vi "parseRangeMode.vi"(8 "error in (no error)":errorcluster, 11 "String":string) -> (0 "error out":errorcluster, 3 "Data":dbl[](array[numeric]))   [LabVIEW 2023, in "CCD.lvclass"]
uses:
  CCD.lvclass
  8fe7bb78-7376-43c1-906c-2fa6ce8d17f9.vi
  <vilib>/JDP Science/JSONtext/Find Item.vi
  <vilib>/JDP Science/JSONtext/Next JSON Value.vi
  <vilib>/JDP Science/JSONtext/String Subset.vi
  <vilib>/JDP Science/JSONtext/Parsing/Advance past next JSON Value (inlined COPY).vi
  <vilib>/JDP Science/JSONtext/Parsing/Advance past whitespace.vi
  <vilib>/JDP Science/JSONtext/Parsing/Advance past String.vi
  <vilib>/JDP Science/JSONtext/Parsing/Advance past Number.vi
  <vilib>/JDP Science/JSONtext/Parsing/Advance past Line Ending.vi
  <vilib>/JDP Science/JSONtext/Parsing/Parse Full Path or Item Name.vi
  <vilib>/JDP Science/JSONtext/Parsing/Advance past Array.vi
  <vilib>/JDP Science/JSONtext/Parsing/Advance past Object.vi
  <vilib>/JDP Science/JSONtext/support/Error Cluster From Code.vi
  <vilib>/JDP Science/JSONtext/Offset/Find Item Locations by Path.vi
  <vilib>/JDP Science/JSONtext/JSON text to Variant.vi
  <vilib>/JDP Science/JSONtext/LVClass Serializer/JSONtext LVClass Serializer.lvclass
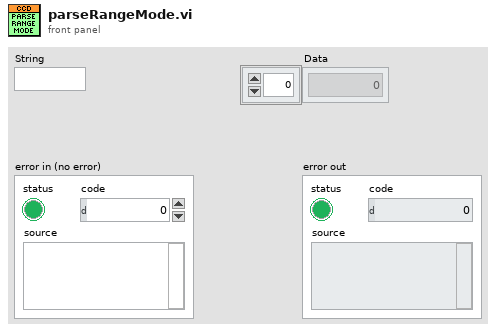
[diagram p1: front panel]
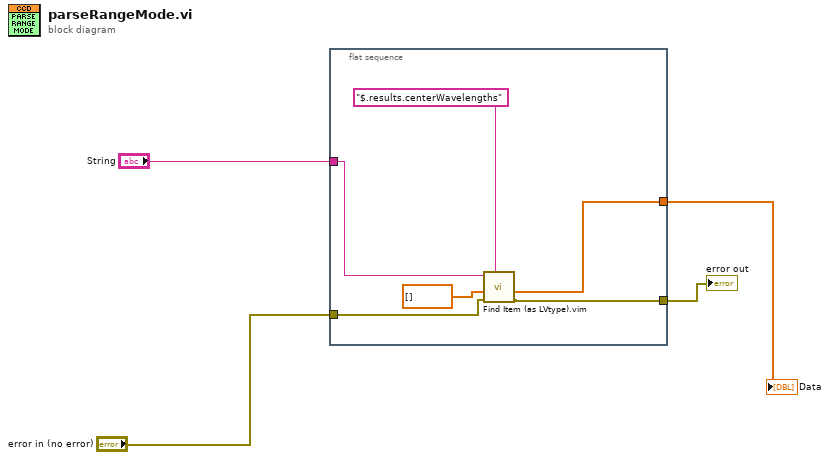
[diagram p0: block diagram]
diagram:
  n1 = flat-sequence {
    tunnel: "String" -> [w9]
    tunnel: [w7] -> w2
    tunnel: "error in (no error)" -> [w6]
    tunnel: [w5] -> w4
    frame #0 {
      n2 = call "Find Item (as LVtype).vim"("$Path or Item Name"="$.results.centerWavelengths", "error in (no error)"=w6, "Data Type and Default Value"=dbl[] [], "JSON"=w9) -> ("error out"=w5:errorcluster, "Data"=w7:dbl[])  [unwired: 4 in, 2 out]
    }
  }
  "error out" <- w4
  "Data" <- w2
